vi "Analog Input - Filtering_v2.vi"() -> ()   [LabVIEW 2021]
doc: "This example demonstrates how to utilize filtering properties of C Series and FieldDAQ devices.\n\nFor instructions on how to connect your signals to the DAQ device, refer to your device documentation."
uses:
  <vilib>/Utility/error.llb/DialogType.ctl
  <vilib>/DAQmx/read.llb/DAQmx Read (Analog 1D Wfm NChan NSamp).vi
  <vilib>/DAQmx/configure/timing.llb/DAQmx Timing (Sample Clock).vi
  <vilib>/DAQmx/configure/task.llb/DAQmx Configure Logging (TDMS).vi
  <vilib>/DAQmx/configure/trigger.llb/DAQmx Start Trigger (Digital Edge).vi
  <vilib>/DAQmx/configure/trigger.llb/DAQmx Start Trigger (Time).vi
  <vilib>/DAQmx/configure/trigger.llb/DAQmx Start Trigger (Analog Edge).vi
  <vilib>/DAQmx/miscellaneous.llb/DAQmx Fill In Error Info.vi
  <resource>/objmgr/daqmx.rc
panel:
  out "P7":dbl[](array[numeric])
  out "P6":dbl[](array[numeric])
  out "P5":dbl[](array[numeric])
  out "P3":dbl[](array[numeric])
  out "P2":dbl[](array[numeric])
  out "P1":dbl[](array[numeric])
  out "P0":dbl[](array[numeric])
  out "Waveform Chart":waveform(dbl)[](graph)
  out "Actual Filter Response":i32(ring)=16152 items=["Comb"=16152, "Bessel"=16153, "Brickwall"=16155, "Butterworth"=16076]
  in  "Filter Response":i32(ring)=16152 items=["Comb"=16152, "Bessel"=16153, "Brickwall"=16155, "Butterworth"=16076]
  out "Actual Filter Order":u32
  in  "Filter Order":u32=1
  out "Actual Filter Frequency":dbl
  in  "Filter Frequency":dbl=1000.0
  in  "Filter":enum16{"No Filtering", "Filtering"}(ring)=enum."Filtering"
  in  "Trigger Type":T1(tab)
  in  "Digital Start Trigger Edge":i32(ring)=10280 caption="Edge" items=["Rising"=10280, "Falling"=10171]
  in  "Digital Start Trigger Source":tag="/Dev1/PFI0" caption="Source"
  in  "Digital Pause Trigger Pause When":i32(ring)=10192 caption="Pause When" items=["High"=10192, "Low"=10214]
  in  "Digital Pause Trigger Source":tag="/Dev1/PFI0" caption="Source"
  in  "Analog Start Trigger Level":dbl caption="Level" format="%0.2f"
  in  "Analog Start Trigger Hysteresis":dbl caption="Hysteresis" format="%.2f"
  in  "Analog Start Trigger Slope":i32(ring)=10280 caption="Slope" items=["Rising"=10280, "Falling"=10171]
  in  "Analog Start Trigger Source":string="APFI0" caption="Source"
  in  "Analog Pause Trigger Source":string="APFI0" caption="Source"
  in  "Analog Pause Trigger Pause When":i32(ring)=10093 caption="Pause When" items=["Above Level"=10093, "Below Level"=10107]
  in  "Analog Pause Trigger Level":dbl caption="Level" format="%.2f"
  in  "When":timestamp
  in  "Select Time\nManually":bool
  in  "Stop":bool
  in  "TDMS File Path":path
  in  "Number of Samples":i32=100
  in  "Sample Rate":dbl=1000.0
  in  "Sample Clock Source":tag="OnboardClock"
  out "Actual Sample Rate":dbl=1000.0 format="%0.2f"
  in  "Logging Mode":i32(ring)=10231 items=["Off"=10231, "Log and Read"=15842]
  # "Channel Settings"
  # "Acquired Data"
  # "Timing Settings"
  # "Trigger Settings"
  # "Logging Settings"
  # "Filtering Settings"
  # "Task Type Settings"
  # "To enable triggers, select a tab above, and configure the settings.\n\nNot all hardware supports all trigger types. Refer to your device documentation for more information."
  # "This trigger type is not supported in continuous sample timing. \n\nRefer to your device documentation for more information on which triggers are supported."
  # "This trigger type is not supported in continuous sample timing. \n\nRefer to your device documentation for more information on which triggers are supported."
  # "If time is not manually set, task will begin after 10 seconds"
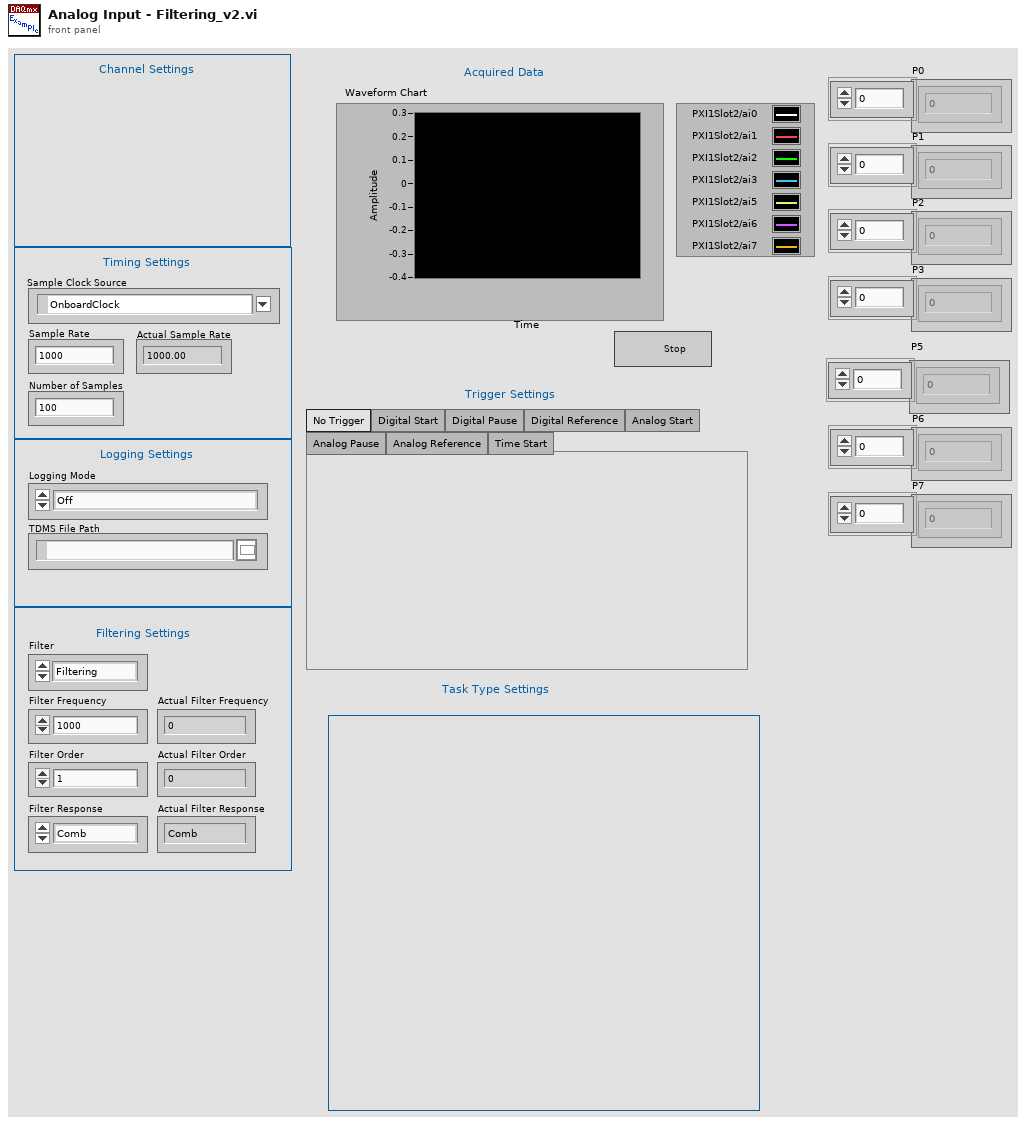
[diagram p1: front panel]
types:
  T1 = enum32{"No Trigger", "Digital Start", "Digital Pause", "Digital Reference", "Analog Start", "Analog Pause", "Analog Reference", "Time Start"}
  T2 = typedef "DialogType.ctl" = u16
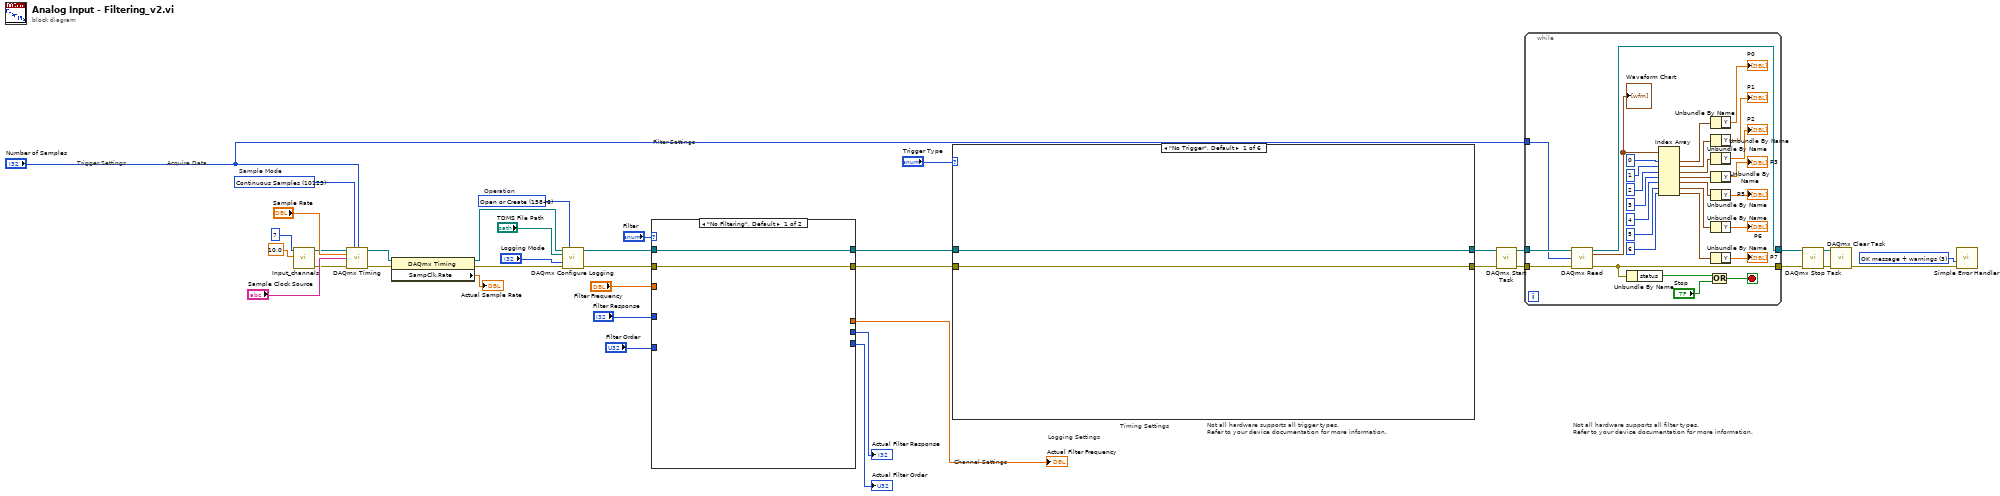
[diagram p0: block diagram]
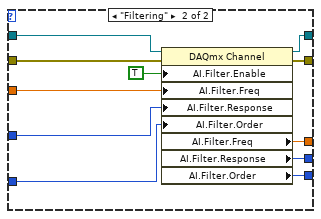
[diagram p2: hidden frame]
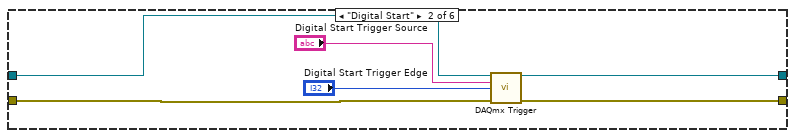
[diagram p3: hidden frame]
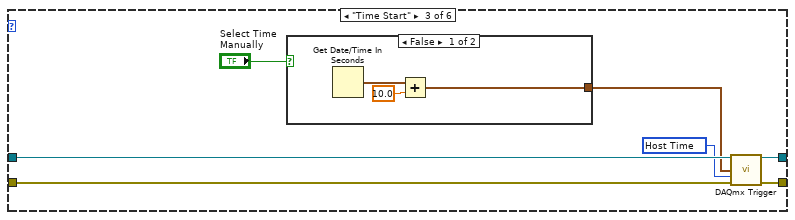
[diagram p4: hidden frame]
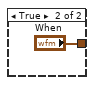
[diagram p5: hidden frame]
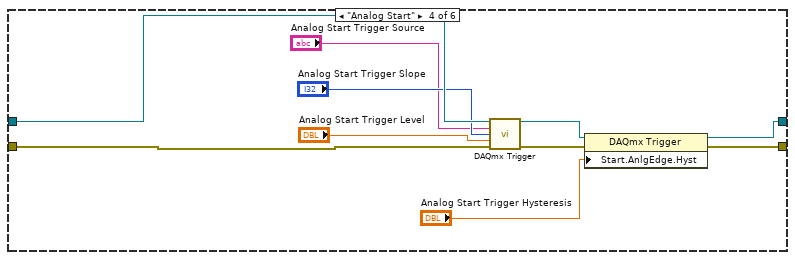
[diagram p6: hidden frame]
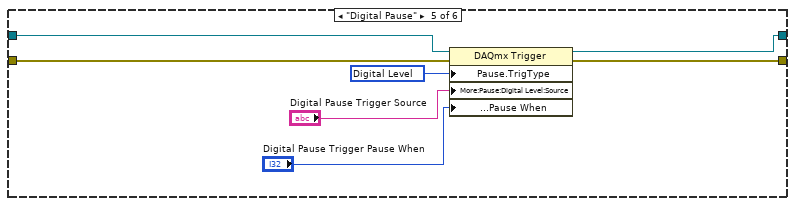
[diagram p7: hidden frame]
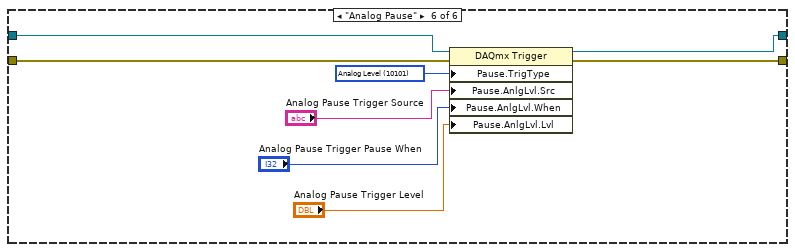
[diagram p8: hidden frame]
diagram:
  w19 = T2 3 items=["no dialog", "OK message", "continue or stop message", "OK message + warnings", "continue/stop + warnings"] ("type of dialog (OK msg:1)")
  w33 = 15846 items=["Open"=10437, "Open or Create"=15846, "Create or Replace"=15847, "Create"=15848]  # Operation
  w36 = 10123 items=["Finite Samples"=10178, "Continuous Samples"=10123, "Hardware Timed Single Point"=12522]  # Sample Mode
  # "Filter Settings"
  # "Not all hardware supports all filter types.\nRefer to your device documentation for more information."
  # "Trigger Settings"
  # "Not all hardware supports all trigger types.\nRefer to your device documentation for more information."
  # "Acquire Data"
  # "Timing Settings"
  # "Channel Settings"
  # "Logging Settings"
  n1 = call "Input_channels.vi"("Range"=10.0, "nchan"=u32 7) -> ("error out"=w3:errorcluster, "Refnum out"=w4:refnum<k21>)  [unwired: 8 in]
  n2 = call-poly <vilib>:"DAQmx Timing.vi"("task/channels in"=w4, "sample mode"=w36, "samples per channel"="Number of Samples", "rate"="Sample Rate", "source"="Sample Clock Source", "error in"=w3) -> ("task out"=w38:refnum<k21>, "error out"=w37:errorcluster)  [unwired: 8 in]
  n3 = property class="DAQmx Timing"(reference=w38, error in=w37) -> (reference out=w35:refnum<k21>, error out=w34:errorcluster, "SampClk.Rate"=→"Actual Sample Rate":dbl)
  n4 = call-poly <vilib>:"DAQmx Configure Logging.vi"("task/channels in"=w35, "operation"=w33, "file path"="TDMS File Path", "logging mode"="Logging Mode", "error in"=w34) -> ("task out"=w14:refnum<k21>, "error out"=w13:errorcluster)  [unwired: 9 in]
  n5 = case shown="\"No Filtering\", Default" "Filter" {
    tunnel: w14 -> [w40 w51]
    tunnel: w13 -> [w39 w48]
    tunnel: [w40 w50] -> w12
    tunnel: [w39 w49] -> w11
    tunnel: "Filter Frequency" -> [_ w47]
    tunnel: "Filter Order" -> [_ w44]
    tunnel: [_ w43] -> w8
    tunnel: [_ w41] -> w7
    tunnel: [_ w42] -> w5
    tunnel: "Filter Response" -> [_ w45]
    frame "No Filtering", Default {
    }
    frame "Filtering" {
      n6 = property class="DAQmx Channel"(reference=w51, error in=w48, "AI.Filter.Enable"=TRUE, "AI.Filter.Freq"=w47, "AI.Filter.Response"=w45, "AI.Filter.Order"=w44) -> (reference out=w50:refnum<k21>, error out=w49:errorcluster, "AI.Filter.Freq"=w43:dbl, "AI.Filter.Response"=w42:i32, "AI.Filter.Order"=w41:u32)
    }
  }
  "Actual Filter Frequency" <- w8
  "Actual Filter Order" <- w7
  "Actual Filter Response" <- w5
  n7 = case shown="\"No Trigger\", Default" "Trigger Type" {
    tunnel: w12 -> [w53 w59 w66 w80 w87 w95]
    tunnel: w11 -> [w52 w58 w65 w79 w84 w92]
    tunnel: [w53 w57 w64 w77 w86 w94] -> w16
    tunnel: [w52 w56 w63 w76 w85 w93] -> w17
    frame "No Trigger", Default {
    }
    frame "Digital Start" {
      n8 = call-poly <vilib>:"DAQmx Trigger.vi"("task/channels in"=w59, "source"="Digital Start Trigger Source", "edge"="Digital Start Trigger Edge", "error in"=w58) -> ("task out"=w57:refnum<k21>, "error out"=w56:errorcluster)  [unwired: 10 in]
    }
    frame "Time Start" {
      w62 = 16126 items=["Host Time"=16126, "I/O Device Time"=16127] ("timescale")
      n9 = case shown="False" "Select Time\nManually" {
        tunnel: [w67 "When"] -> w60
        frame False {
          n10 = Get Date/Time In Seconds() -> (seconds since 1Jan1904=w69:timestamp)
          n11 = Add(x=w69, y=10.0) -> (x+y=w67:timestamp)
        }
        frame True {
        }
      }
      n12 = call-poly <vilib>:"DAQmx Trigger.vi"("task/channels in"=w66, "when"=w60, "timescale"=w62, "error in"=w65) -> ("task out"=w64:refnum<k21>, "error out"=w63:errorcluster)  [unwired: 10 in]
    }
    frame "Analog Start" {
      n13 = call-poly <vilib>:"DAQmx Trigger.vi"("task/channels in"=w80, "source"="Analog Start Trigger Source", "slope"="Analog Start Trigger Slope", "level"="Analog Start Trigger Level", "error in"=w79) -> ("task out"=w75:refnum<k21>, "error out"=w74:errorcluster)  [unwired: 9 in]
      n14 = property class="DAQmx Trigger"(reference=w75, error in=w74, "Start.AnlgEdge.Hyst"="Analog Start Trigger Hysteresis") -> (reference out=w77:refnum<k21>, error out=w76:errorcluster)
    }
    frame "Digital Pause" {
      w83 = 10152 items=["Analog Level"=10101, "Analog Window"=10103, "Digital Level"=10152, "Digital Pattern"=10398, "None"=10230] ("Pause.TrigType")
      n15 = property class="DAQmx Trigger"(reference=w87, error in=w84, "Pause.TrigType"=w83, "More:Pause:Digital Level:Source"="Digital Pause Trigger Source", "More:Pause:Digital Level:Pause When"="Digital Pause Trigger Pause When") -> (reference out=w86:refnum<k21>, error out=w85:errorcluster)
    }
    frame "Analog Pause" {
      w91 = 10101 items=["Analog Level"=10101, "Analog Window"=10103, "Digital Level"=10152, "Digital Pattern"=10398, "None"=10230] ("Pause.TrigType")
      n16 = property class="DAQmx Trigger"(reference=w95, error in=w92, "Pause.TrigType"=w91, "Pause.AnlgLvl.Src"="Analog Pause Trigger Source", "Pause.AnlgLvl.When"="Analog Pause Trigger Pause When", "Pause.AnlgLvl.Lvl"="Analog Pause Trigger Level") -> (reference out=w94:refnum<k21>, error out=w93:errorcluster)
    }
  }
  n17 = call <vilib>:"DAQmx Start Task.vi"("task/channels in"=w16, "error in"=w17) -> ("task out"=w32:refnum<k21>, "error out"=w31:errorcluster)  [unwired: 12 in]
  n18 = while {
    tunnel: w32 -> [w125]
    tunnel: w31 -> [w124]
    tunnel: [w123] -> w23
    tunnel: [w121] -> w22
    tunnel: "Number of Samples" -> [w118]
    stop <- w119 stop-if-true
    n19 = call-poly <vilib>:"DAQmx Read.vi"("task/channels in"=w125, "number of samples per channel"=w118, "error in"=w124) -> ("task out"=w123:refnum<k21>, "data"=w117:waveform(dbl)[], "error out"=w121:errorcluster)  [unwired: 10 in]
    "Waveform Chart" <- w117
    n20 = Unbundle By Name(w121) -> ("status"=w120:bool)
    n21 = Index Array(array=w117, index #1=0 ("index"), index #2=1 ("index"), index #3=2 ("index"), index #4=3 ("index"), index #5=4 ("index"), index #6=5 ("index"), index #7=6 ("index")) -> (element #1=w116:waveform(dbl), element #2=w107:waveform(dbl), element #3=w106:waveform(dbl), element #4=w105:waveform(dbl), element #5=w104:waveform(dbl), element #6=w103:waveform(dbl), element #7=w102:waveform(dbl))
    n22 = Or(x=w120, y="Stop") -> (x .or. y?=w119:bool)
    n23 = Unbundle By Name(w116) -> ("Y"=→"P0":dbl[])
    n24 = Unbundle By Name(w107) -> ("Y"=→"P1":dbl[])
    n25 = Unbundle By Name(w106) -> ("Y"=→"P2":dbl[])
    n26 = Unbundle By Name(w105) -> ("Y"=→"P3":dbl[])
    n27 = Unbundle By Name(w104) -> ("Y"=→"P5":dbl[])
    n28 = Unbundle By Name(w103) -> ("Y"=→"P6":dbl[])
    n29 = Unbundle By Name(w102) -> ("Y"=→"P7":dbl[])
  }
  n30 = call <vilib>:"DAQmx Stop Task.vi"("task/channels in"=w23, "error in"=w22) -> ("task out"=w20:refnum<k21>, "error out"=w21:errorcluster)  [unwired: 12 in]
  n31 = call <vilib>:"DAQmx Clear Task.vi"("task in"=w20, "error in"=w21) -> ("error out"=w30:errorcluster)  [unwired: 13 in]
  n32 = call <vilib>:"Simple Error Handler.vi"("type of dialog (OK msg:1)"=w19, "error in (no error)"=w30) -> ()  [unwired: 3 in, 5 out]
